vi "ConfigUtilities - Init Tx Packet Page.vi"(7 "Tx Packets Cluster In":T1, 8 "error in (no error)":errorcluster, 11 "Node Ptr In":T2 format="%.0x") -> (0 "error out":errorcluster, 3 "Node Ptr Out":T2 format="%.0x", 5 "Tx Packets Cluster Out":T1)   [LabVIEW 2016, in "UDP-Custom-Device System Explorer.lvlib"]
uses:
  UDP-Custom-Device System Explorer.lvlib
  <vilib>/NI Veristand/Custom Device API/Custom Device Item Ref.ctl
  Types/TypeDef - Tx Packets Page References.ctl
  Shared/Constants.vi
  <vilib>/NI Veristand/Custom Device API/Get Item Property (Boolean).vi
  <vilib>/NI Veristand/Custom Device API/Get Item Property (I32).vi
  <vilib>/NI Veristand/Custom Device API/Get Item Property (String).vi
  <vilib>/NI Veristand/Custom Device API/Get Item Property (U32).vi
  <vilib>/NI VeriStand/Custom Device API/Custom Device API.lvlib
  Shared/UDP-Custom-Device Shared.lvlib
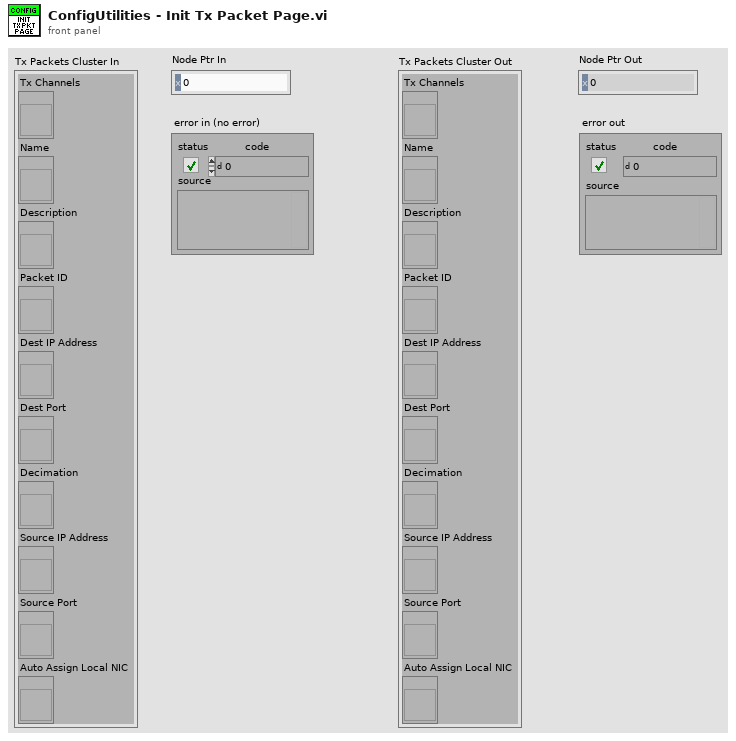
[diagram p1: front panel]
types:
  T1 = typedef "UDP-Custom-Device System Explorer.lvlib/TypeDef - Tx Packets Page References.ctl" = cluster{"Tx Channels":refnum<vi>, "Name":refnum<vi>, "Description":refnum<vi>, "Packet ID":refnum<vi>, "Dest IP Address":refnum<vi>, "Dest Port":refnum<vi>, "Decimation":refnum<vi>, "Source IP Address":refnum<vi>, "Source Port":refnum<vi>, "Auto Assign Local NIC":refnum<vi>}
  T2 = typedef "Custom Device API.lvlib/Custom Device Item Ref.ctl" = u64
  T3 = typedef "Custom Device API.lvlib/Custom Device Item Info.ctl" = cluster{"Name":string, "Is Channel":bool, "GUID":string, "Is Waveform":bool}
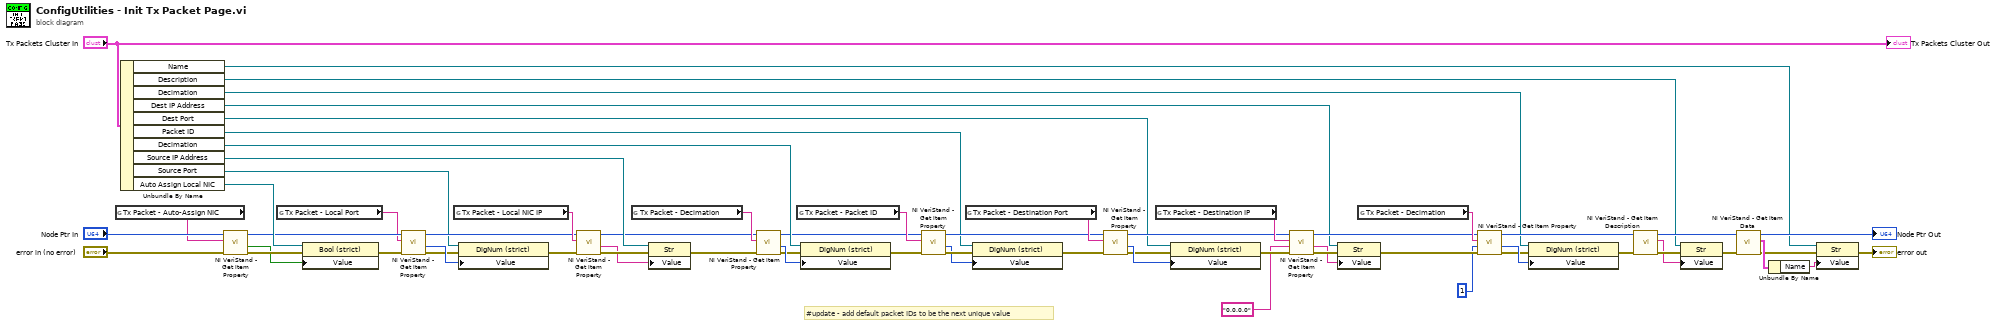
[diagram p0: block diagram]
diagram:
  # "#update - add default packet IDs to be the next unique value"
  n1 = global read "Constants.vi" "Tx Packet - Auto-Assign NIC"() -> (w1:string)
  n2 = Unbundle By Name("Tx Packets Cluster In") -> ("Name"=w26:refnum<vi>, "Description"=w27:refnum<vi>, "Decimation"=w31:refnum<vi>, "Dest IP Address"=w32:refnum<vi>, "Dest Port"=w33:refnum<vi>, "Packet ID"=w34:refnum<vi>, "Decimation"=w24:refnum<vi>, "Source IP Address"=w20:refnum<vi>, "Source Port"=w11:refnum<vi>, "Auto Assign Local NIC"=w6:refnum<vi>)
  n3 = call-poly <vilib>:"NI VeriStand - Get Item Property.vi"("error in (no error)"="error in (no error)", "Property Name"=w1, "Item Ref in"="Node Ptr In") -> ("error out"=w7:errorcluster, "Value"=w2:bool, "Item Ref out"=w5:T2)  [unwired: 5 in, 1 out]
  n4 = global read "Constants.vi" "Tx Packet - Local Port"() -> (w3:string)
  n5 = property class="Bool (strict)"(reference=w6, error in=w7, "Value"=w2) -> (error out=w4:errorcluster)  [unwired: 1 out]
  n6 = call-poly <vilib>:"NI VeriStand - Get Item Property.vi"("error in (no error)"=w4, "Property Name"=w3, "Item Ref in"=w5) -> ("error out"=w8:errorcluster, "Value"=w10:i32, "Item Ref out"=w13:T2)  [unwired: 5 in, 1 out]
  n7 = global read "Constants.vi" "Tx Packet - Local NIC IP"() -> (w14:string)
  n8 = property class="DigNum (strict)"(reference=w11, error in=w8, "Value"=w10) -> (error out=w9:errorcluster)  [unwired: 1 out]
  n9 = call-poly <vilib>:"NI VeriStand - Get Item Property.vi"("error in (no error)"=w9, "Property Name"=w14, "Item Ref in"=w13) -> ("error out"=w18:errorcluster, "Value"=w17:string, "Item Ref out"=w12:T2)  [unwired: 5 in, 1 out]
  n10 = global read "Constants.vi" "Tx Packet - Decimation"() -> (w22:string)
  n11 = property class="Str"(reference=w20, error in=w18, "Value"=w17) -> (error out=w21:errorcluster)  [unwired: 1 out]
  n12 = call-poly <vilib>:"NI VeriStand - Get Item Property.vi"("error in (no error)"=w21, "Property Name"=w22, "Item Ref in"=w12) -> ("error out"=w16:errorcluster, "Value"=w23:u32, "Item Ref out"=w15:T2)  [unwired: 5 in, 1 out]
  n13 = global read "Constants.vi" "Tx Packet - Packet ID"() -> (w61:string)
  n14 = property class="DigNum (strict)"(reference=w24, error in=w16, "Value"=w23) -> (error out=w19:errorcluster)  [unwired: 1 out]
  n15 = call-poly <vilib>:"NI VeriStand - Get Item Property.vi"("error in (no error)"=w19, "Property Name"=w61, "Item Ref in"=w15) -> ("error out"=w60:errorcluster, "Value"=w59:i32, "Item Ref out"=w52:T2)  [unwired: 5 in, 1 out]
  n16 = global read "Constants.vi" "Tx Packet - Destination Port"() -> (w56:string)
  n17 = property class="DigNum (strict)"(reference=w34, error in=w60, "Value"=w59) -> (error out=w50:errorcluster)  [unwired: 1 out]
  n18 = call-poly <vilib>:"NI VeriStand - Get Item Property.vi"("error in (no error)"=w50, "Property Name"=w56, "Item Ref in"=w52) -> ("error out"=w57:errorcluster, "Value"=w58:i32, "Item Ref out"=w51:T2)  [unwired: 5 in, 1 out]
  n19 = global read "Constants.vi" "Tx Packet - Destination IP"() -> (w55:string)
  n20 = property class="DigNum (strict)"(reference=w33, error in=w57, "Value"=w58) -> (error out=w49:errorcluster)  [unwired: 1 out]
  n21 = call-poly <vilib>:"NI VeriStand - Get Item Property.vi"("error in (no error)"=w49, "Default Value"="0.0.0.0", "Property Name"=w55, "Item Ref in"=w51) -> ("error out"=w54:errorcluster, "Value"=w53:string, "Item Ref out"=w45:T2)  [unwired: 4 in, 1 out]
  n22 = property class="Str"(reference=w32, error in=w54, "Value"=w53) -> (error out=w44:errorcluster)  [unwired: 1 out]
  n23 = global read "Constants.vi" "Tx Packet - Decimation"() -> (w46:string)
  n24 = call-poly <vilib>:"NI VeriStand - Get Item Property.vi"("error in (no error)"=w44, "Default Value"=1, "Property Name"=w46, "Item Ref in"=w45) -> ("error out"=w47:errorcluster, "Value"=w48:i32, "Item Ref out"=w43:T2)  [unwired: 4 in, 1 out]
  n25 = property class="DigNum (strict)"(reference=w31, error in=w47, "Value"=w48) -> (error out=w42:errorcluster)  [unwired: 1 out]
  n26 = call <vilib>:"NI VeriStand - Get Item Description.vi"("error in (no error)"=w42, "Item Ref in"=w43) -> ("error out"=w41:errorcluster, "Description"=w40:string, "Item Ref out"=w38:T2)  [unwired: 7 out]
  n27 = property class="Str"(reference=w27, error in=w41, "Value"=w40) -> (error out=w39:errorcluster)  [unwired: 1 out]
  n28 = call <vilib>:"NI VeriStand - Get Item Data.vi"("error in (no error)"=w39, "Item Ref in"=w38) -> ("error out"=w63:errorcluster, "Item Info"=w64:T3, "Item Ref out"=→"Node Ptr Out":T2)  [unwired: 6 in, 1 out]
  n29 = Unbundle By Name(w64) -> ("Name"=w37:string)
  n30 = property class="Str"(reference=w26, error in=w63, "Value"=w37) -> (error out=→"error out":errorcluster)  [unwired: 1 out]
  "Tx Packets Cluster Out" <- "Tx Packets Cluster In"
